vi "MeasureRMS.vi"(2 "Sampling Rate":dbl, 3 "# of Samples":dbl) -> (0 "Waveform Graph":dynamicdata(graph), 1 "RMS":dbl)   [LabVIEW 2015]
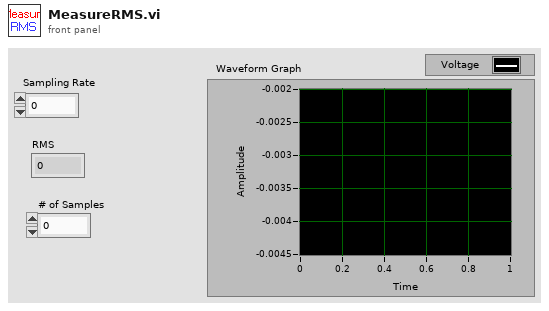
[diagram p1: front panel]
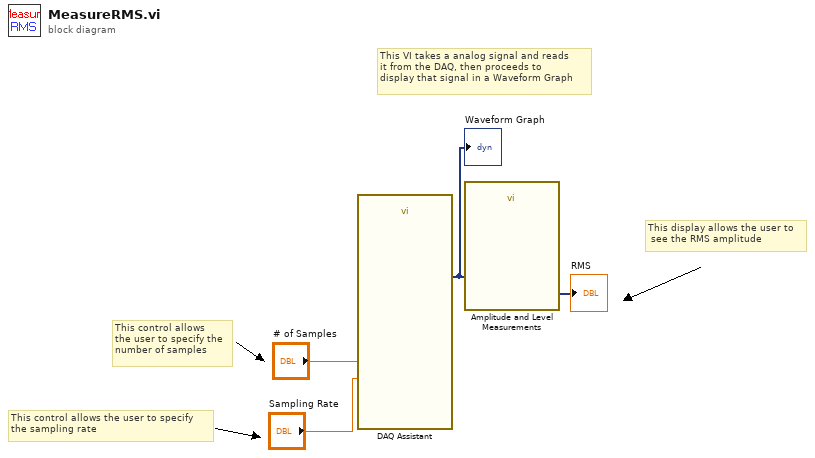
[diagram p0: block diagram]
diagram:
  # "This display allows the user to\n see the RMS amplitude"
  # "This control allows the user to specify \nthe sampling rate"
  # "This control allows\nthe user to specify the\nnumber of samples"
  # "This VI takes a analog signal and reads\nit from the DAQ, then proceeds to \ndisplay that signal in a Waveform Graph"
  n1 = call "DAQ Assistant"("rate"="Sampling Rate", "number of samples"="# of Samples") -> ("data"=w1:dynamicdata)  [unwired: 15 in, 2 out]
  "Waveform Graph" <- w1
  n2 = call "Amplitude and Level Measurements"("Signals"=w1) -> ("RMS"=→"RMS":dynamicdata)  [unwired: 13 in, 1 out]
